vi "PSDS_Destroy Object.vi"(8 "error in (no error)":errorcluster, 11 "Object Name":string) -> (0 "error out":errorcluster)   [LabVIEW 2016]
panel:
  # "Data Out"
  # "Data In"
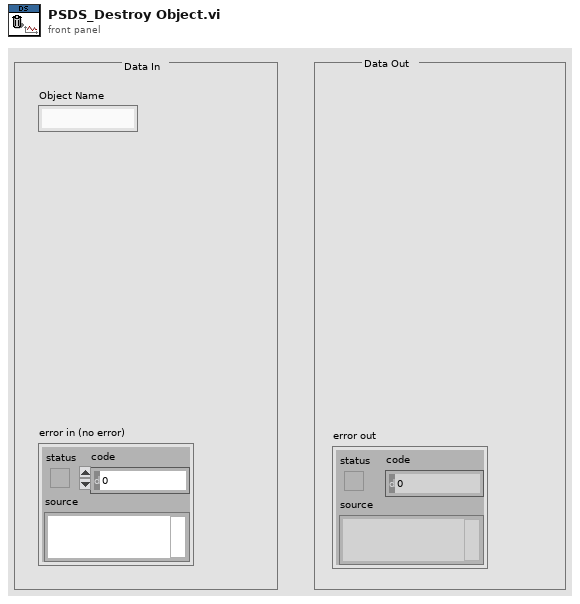
[diagram p1: front panel]
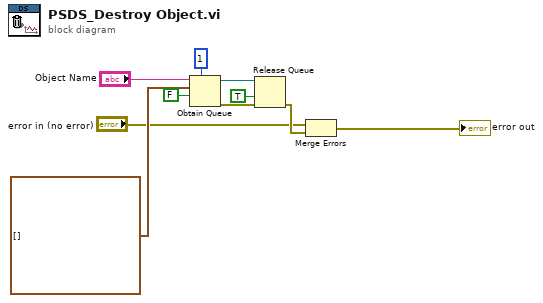
[diagram p0: block diagram]
diagram:
  n1 = Obtain Queue(max queue size (-1, unlimited)=1 ("队列最大值（-1，无限）"), name (unnamed)="Object Name", element data type=waveform(dbl)[] [] ("Wave"), create if not found? (T)=FALSE ("如未找到是否创建？(T)")) -> (queue out=w9:refnum<queue>, error out=w8:errorcluster)  [unwired: 1 in, 1 out]
  n2 = Release Queue(queue=w9, force destroy? (F)=TRUE ("强制销毁？(F)"), error in (no error)=w8) -> (error out=w4:errorcluster)  [unwired: 2 out]
  n3 = Merge Errors("error in (no error)", w4) -> (→"error out":errorcluster)
